vi "classInvenventory.vi"(8 "error in":errorcluster) -> (0 "error out":errorcluster, 1 "ILabelableList":refnum<class "ILabelable.lvclass">[](array[class]), 2 "ICreatableList":refnum<class "ICreatable.lvclass">[](array[class]), 3 "classList":refnum<class "Generic.lvclass">[](array[class]))   [LabVIEW 2023, in "TLC_Scripto.lvlib"]
uses:
  TLC_Scripto.lvlib
  Generic/Generic.lvclass
  ILabelable/ILabelable.lvclass
  ICreatable/ICreatable.lvclass
  GObject/GObject.lvclass
  Control/Control.lvclass
  Decoration/Decoration.lvclass
  TextDecoration/TextDecoration.lvclass
  Wire/Wire.lvclass
  BlockDiagram/BlockDiagram.lvclass
  Terminal/Terminal.lvclass
  ControlTerminal/ControlTerminal.lvclass
  Node/Node.lvclass
  Structure/Structure.lvclass
  C:/projects/TLC_Scripto/Source/Generic/Generic.lvclass
  C:/projects/TLC_Scripto/Source/GObject/GObject.lvclass
  C:/projects/TLC_Scripto/Source/Control/Control.lvclass
  C:/projects/TLC_Scripto/Source/Decoration/Decoration.lvclass
  C:/projects/TLC_Scripto/Source/ICreatable/ICreatable.lvclass
  C:/projects/TLC_Scripto/Source/Wire/Wire.lvclass
  C:/projects/TLC_Scripto/Source/ILabelable/ILabelable.lvclass
  C:/projects/TLC_Scripto/Source/TextDecoration/TextDecoration.lvclass
  C:/projects/TLC_Scripto/Source/BlockDiagram/BlockDiagram.lvclass
  C:/projects/TLC_Scripto/Source/Terminal/Terminal.lvclass
  C:/projects/TLC_Scripto/Source/ControlTerminal/ControlTerminal.lvclass
  C:/projects/TLC_Scripto/Source/Node/Node.lvclass
  C:/projects/TLC_Scripto/Source/Structure/Structure.lvclass
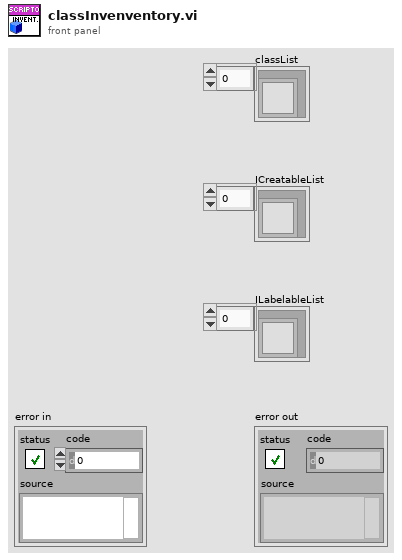
[diagram p1: front panel]
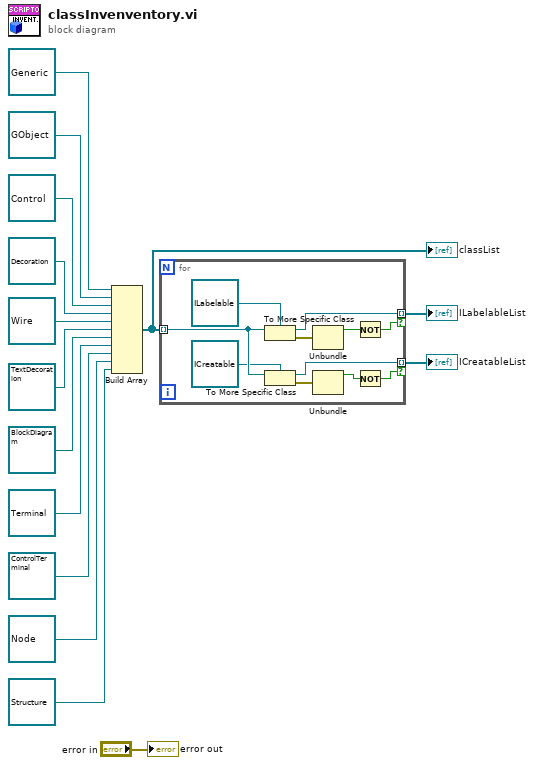
[diagram p0: block diagram]
diagram:
  n1 = Build Array(refnum<class "Generic.lvclass"> refnum ("TLC_Scripto.lvlib:GObject"), refnum<class "GObject.lvclass"> refnum ("TLC_Scripto.lvlib:GObject 2"), refnum<class "Control.lvclass"> refnum ("TLC_Scripto.lvlib:Control.lvclass"), refnum<class "Decoration.lvclass"> refnum ("TLC_Scripto.lvlib:Wire"), refnum<class "Wire.lvclass"> refnum ("TLC_Scripto.lvlib:Wire 2"), refnum<class "TextDecoration.lvclass"> refnum ("TLC_Scripto.lvlib:TextDecoration"), refnum<class "BlockDiagram.lvclass"> refnum ("TLC_Scripto.lvlib:BlockDiagram.lvclass"), refnum<class "Terminal.lvclass"> refnum ("TLC_Scripto.lvlib:Terminal"), refnum<class "ControlTerminal.lvclass"> refnum ("TLC_Scripto.lvlib:ControlTerminal"), refnum<class "Node.lvclass"> refnum ("TLC_Scripto.lvlib:Node"), refnum<class "Structure.lvclass"> refnum ("TLC_Scripto.lvlib:Structure")) -> (w15:refnum<class "Generic.lvclass">[])
  "classList" <- w15
  n2 = for {
    tunnel: w15 -> [w21] mode=indexing
    tunnel: [w25] -> w14 mode=indexing if=w22
    tunnel: [w17] -> w13 mode=indexing if=w16
    n3 = To More Specific Class(target class=refnum<class "ILabelable.lvclass"> refnum ("TLC_Scripto.lvlib:ILabelable.lvclass"), reference=w21) -> (specific class reference=w25:refnum<class "ILabelable.lvclass">, error out=w24:errorcluster)  [unwired: 1 in]
    n4 = To More Specific Class(target class=refnum<class "ICreatable.lvclass"> refnum ("TLC_Scripto.lvlib:ICreatable.lvclass"), reference=w21) -> (specific class reference=w17:refnum<class "ICreatable.lvclass">, error out=w18:errorcluster)  [unwired: 1 in]
    n5 = Unbundle(w24) -> ("status"=w23:bool)  [unwired: 2 out]
    n6 = Unbundle(w18) -> ("status"=w19:bool)  [unwired: 2 out]
    n7 = Not(x=w23) -> (.not. x?=w22:bool)
    n8 = Not(x=w19) -> (.not. x?=w16:bool)
  }
  "ILabelableList" <- w14
  "ICreatableList" <- w13
  "error out" <- "error in"
